vi "sv_Level with IC (equal conf, linear, exp, peak).vi"(0 "scaled signal [EU]":dbl[](array[numeric]) format="%.2f", 1 "sampling frequency [Hz]":dbl=10000.0 format="%.2f", 2 "exponential mode":enum16{"Slow", "Fast", "Impulse", "Custom"}(ring)=enum."Fast", 3 "initial filter state":T1 {"peak detector" format="%.2f"; "exponential averaging" format="%.2f"}, 4 "time constant [ms]":dbl=125.0 min=0.0 format="%.2f", 5 "initial internal state":cluster{"squared sum":dbl, "size":dbl} {"size" format="%.2f"; "squared sum" format="%.2f"}, 6 "averaging type":T2(ring), 7 "init/cont (init:F)":bool, 8 "BT":dbl format="%.2f", 9 "bandwidth [Hz]":dbl format="%.2f") -> (13 "actual time constant [ms]":dbl, 14 "[EU^2 rms] (final value)":dbl, 16 "final filter state":T1, 19 "final internal state":cluster{"squared sum":dbl, "size":dbl})   [LabVIEW 2017, in "SoundVib_Octave_2014 standard.lvlib"]
uses:
  <vilib>/addons/Sound and Vibration/svt_Octave/SoundVib_Octave_2014 standard.lvlib
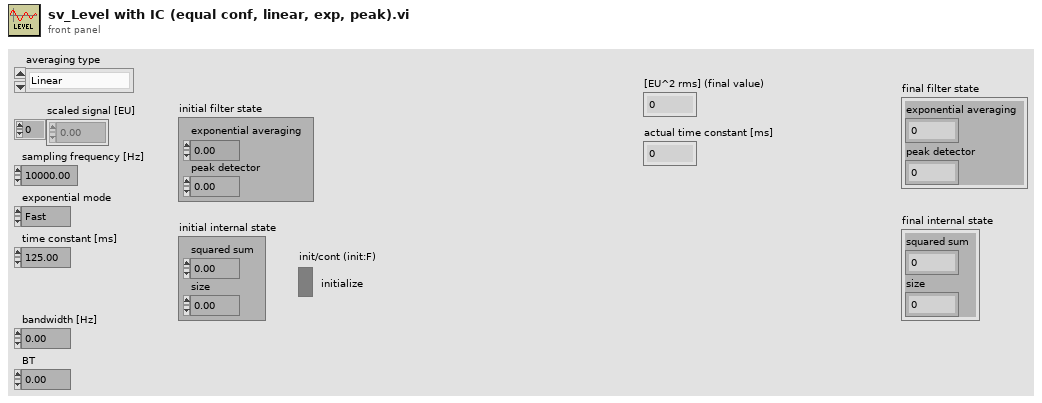
[diagram p1: front panel]
types:
  T1 = cluster{"exponential averaging":dbl, "peak detector":dbl}
  T2 = enum16{"Linear", "Exponential", "Equal confidence", "Peak"}
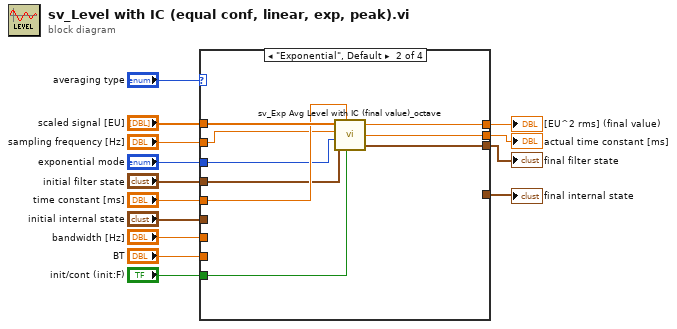
[diagram p0: block diagram]
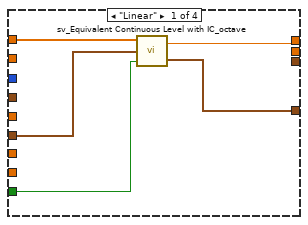
[diagram p2: hidden frame]
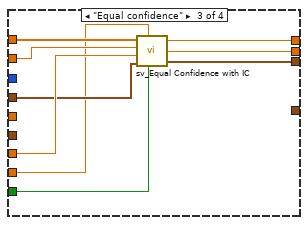
[diagram p3: hidden frame]
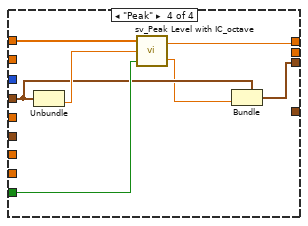
[diagram p4: hidden frame]
diagram:
  n1 = case shown="\"Exponential\", Default" "averaging type" {
    tunnel: "scaled signal [EU]" -> [w19 w28 w37 w44]
    tunnel: "time constant [ms]" -> [_ w27 _ _]
    tunnel: "sampling frequency [Hz]" -> [_ w26 w36 _]
    tunnel: "exponential mode" -> [_ w25 _ _]
    tunnel: "initial filter state" -> [_ w24 w32 w40]
    tunnel: [w15 w23 w35 w42] -> w7
    tunnel: [_ w22 w34 _] -> w6
    tunnel: [_ w21 w29 w38] -> w5
    tunnel: "init/cont (init:F)" -> [w17 w20 w31 w43]
    tunnel: "initial internal state" -> [w18 _ _ _]
    tunnel: [w16 _ _ _] -> w3
    tunnel: "bandwidth [Hz]" -> [_ _ w33 _]
    tunnel: "BT" -> [_ _ w30 _]
    frame "Linear" {
      n2 = call <vilib>:"sv_Equivalent Continuous Level with IC_octave.vi"("init/cont (init:F)"=w17, "initial internal state"=w18, "scaled signal [EU]"=w19) -> ("final internal state"=w16:cluster{"squared sum":dbl, "size":dbl}, "equivalent continuous level [EU^2 rms]"=w15:dbl)
    }
    frame "Exponential", Default {
      n3 = call <vilib>:"sv_Exp Avg Level with IC (final value)_octave.vi"("scaled signal [EU]"=w28, "time constant [ms]"=w27, "sampling frequency [Hz]"=w26, "exponential mode"=w25, "init/cont (init:F)"=w20, "initial filter state"=w24) -> ("exp avg [EU^2 rms] (final value)"=w23:dbl, "actual time constant [ms]"=w22:dbl, "final filter state"=w21:T1)
    }
    frame "Equal confidence" {
      n4 = call <vilib>:"sv_Equal Confidence with IC.vi"("scaled signal [EU]"=w37, "BT"=w30, "sampling frequency [Hz]"=w36, "bandwidth [Hz]"=w33, "init/cont (init:F)"=w31, "initial filter state"=w32) -> ("exp avg [EU^2 rms] (final value)"=w35:dbl, "time constant [ms]"=w34:dbl, "final filter state"=w29:T1)
    }
    frame "Peak" {
      n5 = Unbundle(w40) -> ("peak detector"=w41:dbl)  [unwired: 1 out]
      n6 = call <vilib>:"sv_Peak Level with IC_octave.vi"("init/cont (init:F)"=w43, "initial peak level"=w41, "scaled signal [EU]"=w44) -> ("final peak level"=w39:dbl, "peak level"=w42:dbl)
      n7 = Bundle(cluster=w40, "peak detector"=w39) -> (w38:T1)  [unwired: 1 in]
    }
  }
  "[EU^2 rms] (final value)" <- w7
  "actual time constant [ms]" <- w6
  "final filter state" <- w5
  "final internal state" <- w3
